vi "Read File+ [I16].vi"(6 "2D number of columns/1D count":i32, 7 "2D number of rows":i32, 8 "error in (no error)":errorcluster, 9 "pos offset (bytes:0)":i32, 10 "pos mode (rel. to current:2)":enum16{"start", "end", "current"}(ring)=enum."current", 11 "refnum":refnum<file>) -> (0 "error out":errorcluster, 1 "mark after read (bytes)":i32, 2 "1D data":i16[](array[numeric]), 3 "2D data":i16[][](array[numeric]), 4 "EOF?":bool, 5 "dup refnum":refnum<file>)   [LabVIEW 2009]
doc: "Reads a 2D or 1D array of signed word integers (I16) from a byte stream file at the specified location; the default location is at the current mark. The VI does incoming and internal error checking and does not read if an incoming error occurs.\n\nrefnum is the reference number of the open file.\n\npos mode specifies where the write begins relative to pos offset:\n\n 0: at the beginning of the file plus pos offset.\n\n 1: at the end of the file plus pos offset. \n\n 2: at the current file mark plus pos offset. This is the default value.\n\npos offset specifies in bytes how far from the location specified by pos mode that the operation begins. The default value is 0. Byte units rather than integer (2 byte) units for flexibility, for example, so that a file can contain a text header written with Write File+ (string) followed by arrays of number written with Write File+ [I16].\n\n2D number of rows is the number of rows to create if the data is to be returned in the 2D array output. If the value is 0 (default), the data is returned in the 1D array.\n\n2D number of columns/1D count is the number of columns to create if the data is to be returned in the 2D array output, provided that 2D number of rows is >0; otherwise, this is the number of signed word integers to read and return in the 1D array output.\n\nerror in is a cluster of three elements (error?, code, and source) that describe the upstream error state, that is, the existance of any error preceeding the execution of the VI. The VI executes normally only if no incoming error exists; otherwise it merely passes the error in value to error out. error? is TRUE if an error occurred; the default value is FALSE. code is the error code; the default value is 0. source is in most cases the name of the VI or function that produced the error; the default value is an empty string.\n\ndup refnum is a flow-though parameter with the same value as refnum.\n\n2D array contains the signed word integers read from the file if 2D number of rows is greater than 0; otherwise, this output is empty.\n\n1D array contains the signed word integers read from the file if 2D number of rows equal 0; otherwise, this output is empty.\n\nmark after read is the location of the file mark after the read; it points to the byte in the file following the last byte read.\n\nEOF? is TRUE if you attempt to read past the end of file.\n\nerror out is a cluster of three elements (error?, code, and source) that describe the error state following the execution of the VI. If an incoming error does not exist, the VI executes normally and error out describes the VI's error state; if an incoming error exists, error out equals error in."
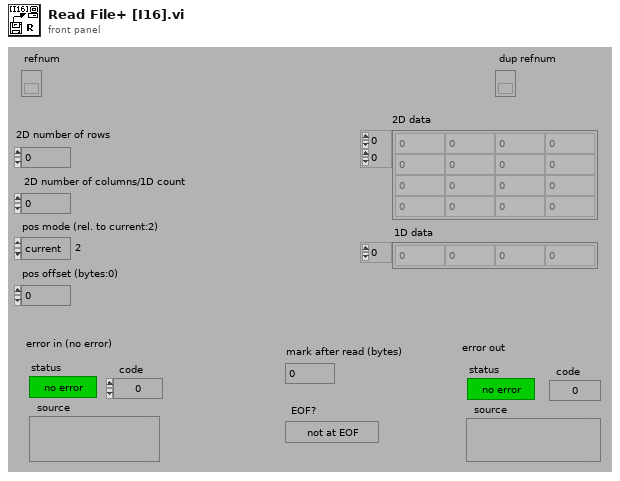
[diagram p1: front panel]
types:
  T1 = cluster{"2D number of rows":i32, "2D number of columns/1D count":i32}
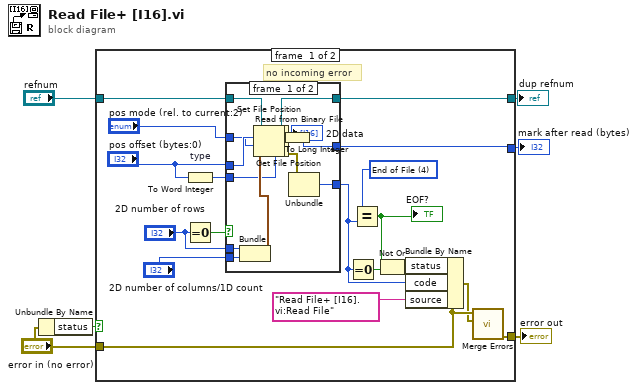
[diagram p0: block diagram]
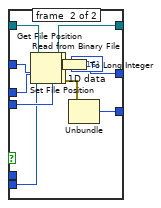
[diagram p2: hidden frame]
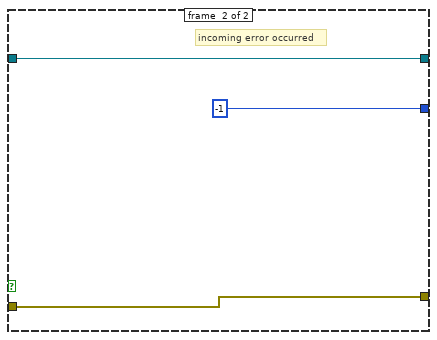
[diagram p3: hidden frame]
diagram:
  n1 = Unbundle By Name("error in (no error)") -> ("status"=w6:bool)
  n2 = case shown="False" w6 {
    tunnel: [w9 w58] -> w5
    tunnel: [w17 -1] -> w4
    tunnel: [w22 w57] -> w3
    tunnel: "refnum" -> [w21 w57]
    tunnel: "error in (no error)" -> [w8 w58]
    frame #0 {
      w11 = 4 items=["No Error", "Manager Argument Error", "Memory Full", "Out of Zone", "End of File", "File Already Open", "Generic File IO Error", "File Not Found", "File Permission Error", "Disk Full", "Duplicate Path", "Too Many Files Open", "Not Enabled", "Resource File Not Found", "Cannot Add Resource", "Resource Not Found", "Image Not Found", "Image Memory Error", "Pen Does Not Exist", "Config Bad Type", "Config Token Not Found", "Config Parse Error", "Config Memory Error", "Bad External Code Format", "Bad External Code Offset", "External Code Not Present", "Null Window", "Destroy Window Mixup", "Null Menu", "Print Aborted", "Bad Print Record", "Print Driver Error", "Windows Error During Print", "Memory Error During Print", "Print Dialog Error", "Generic Print Error", "Invalid Device Refnum", "Device Not Found", "Device Parameter Error", "Device Unit Error", "Can't Open Device", "Device Call Aborted", "Generic Error", "Cancelled By User", "Object ID Too Low", "Object ID Too High", "Object Not In Heap", "Unknown Heap", "Bad DefProc ID", "DefProc Not In Table", "Message Out Of Range", "Null Method", "Unknown Message", "Manager Call Not Supported"]
      # "no incoming error"
      n3 = To Word Integer "type"(number="pos offset (bytes:0)") -> (16bit integer=w24:i16)
      n4 = Equal To 0?(x="2D number of rows") -> (x = 0?=w23:bool)
      n5 = case shown="True" w23 {
        tunnel: [w32 w49] -> w13
        tunnel: [w36 w56] -> w17
        tunnel: w24 -> [w40 w55]
        tunnel: "2D number of columns/1D count" -> [w39 w50]
        tunnel: "2D number of rows" -> [w38 _]
        tunnel: [w35 w52] -> w22
        tunnel: w21 -> [w34 w53]
        tunnel: "pos mode (rel. to current:2)" -> [w30 w47]
        tunnel: "pos offset (bytes:0)" -> [w33 w51]
        frame #0 {
          n6 = Bundle("2D number of rows"=w38, "2D number of columns/1D count"=w39) -> (w41:T1)  [unwired: 1 in]
          n7 = Set File Position(offset (in bytes) (0)=w33, refnum=w34, from (0:start)=w30) -> (refnum out=w29:refnum<file>, error out=w28:errorcluster)  [unwired: 1 in]
          n8 = Read from Binary File(5:w40, 8:w28, 10:w41, 11:w29) -> (0:w26:errorcluster, 2:→"2D data":i16[][], 3:w27:refnum<file>)  [unwired: 2 in, 1 out]
          n9 = Get File Position(4:w26, 7:w27) -> (0:w31:errorcluster, 2:w25:i64, 3:w35:refnum<file>)
          n10 = To Long Integer(number=w25) -> (32bit integer=w36:i32)
          n11 = Unbundle(w31) -> ("code"=w32:i32)  [unwired: 2 out]
        }
        frame #1 {
          n12 = Set File Position(offset (in bytes) (0)=w51, refnum=w53, from (0:start)=w47) -> (refnum out=w46:refnum<file>, error out=w45:errorcluster)  [unwired: 1 in]
          n13 = Read from Binary File(5:w55, 8:w45, 10:w50, 11:w46) -> (0:w43:errorcluster, 2:→"1D data":i16[], 3:w44:refnum<file>)  [unwired: 2 in, 1 out]
          n14 = Get File Position(4:w43, 7:w44) -> (0:w48:errorcluster, 2:w42:i64, 3:w52:refnum<file>)
          n15 = To Long Integer(number=w42) -> (32bit integer=w56:i32)
          n16 = Unbundle(w48) -> ("code"=w49:i32)  [unwired: 2 out]
        }
      }
      n17 = Equal To 0?(x=w13) -> (x = 0?=w15:bool)
      n18 = Equal?(x=w11, y=w13) -> (x = y?=w14:bool)
      "EOF?" <- w14
      n19 = Not Or(1:w15, 2:w14) -> (0:w10:bool)
      n20 = Bundle By Name(cluster=w8, "status"=w10, "code"=w13, "source"="Read File+ [I16].vi:Read File") -> (w7:errorcluster)
      n21 = call <vilib>:"Merge Errors.vi"("error in 2 (no error)"=w7, "error in 1 (no error)"=w8) -> ("error out"=w9:errorcluster)  [unwired: 5 in]
    }
    frame #1 {
      # "incoming error occurred"
    }
  }
  "error out" <- w5
  "mark after read (bytes)" <- w4
  "dup refnum" <- w3
